vi "ConduccionTermica.vi"() -> ()   [LabVIEW 2024]
uses:
  <vilib>/express/express shared/transition.llb/Dynamic To Waveform Array.vi
  <vilib>/express/express signal manip/GetorSetDDTAttributes/Set DDT Attributes/SetT0.vi
  <vilib>/express/express shared/transition.llb/Waveform Array To Dynamic.vi
  <vilib>/express/express signal manip/GetorSetDDTAttributes/Set DDT Attributes/Set DDT Properties.xnode
  <instrlib>/Arduino UNO/Arduino UNO.lvlib
panel:
  out "Sensor V 2":dbl
  out "Sensor 2":string
  out "Temperatura V 5":dbl
  out "Temperatura 5":string
  out "Temperatura V 4":dbl
  out "Temperatura 4":string
  out "Sensor V 1":dbl
  out "Sensor 1":string
  in  "COM 2":refnum<visa-resource-name>
  out "Temperatura V 3":dbl
  out "Temperatura V 2":dbl
  out "Temperatura V 1":dbl
  in  "stop":bool
  in  "COM 1":refnum<visa-resource-name>
  out "Temperatura 3":string
  out "Temperatura 2":string
  out "Temperatura 1":string
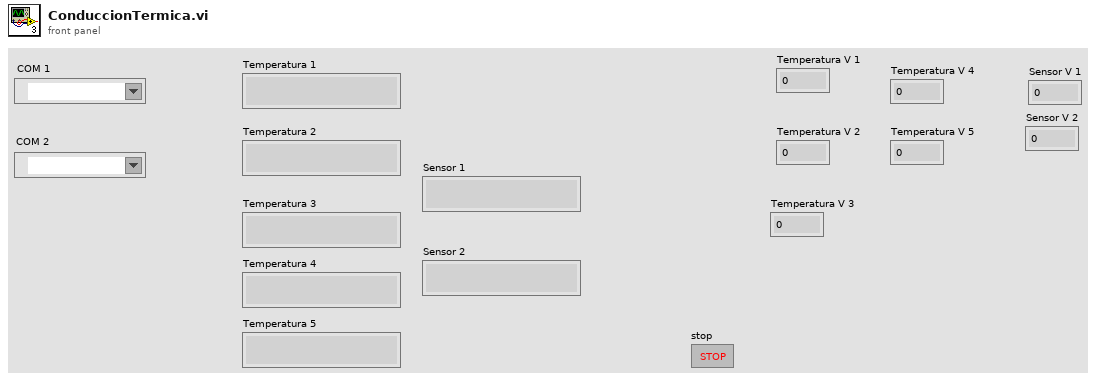
[diagram p1: front panel]
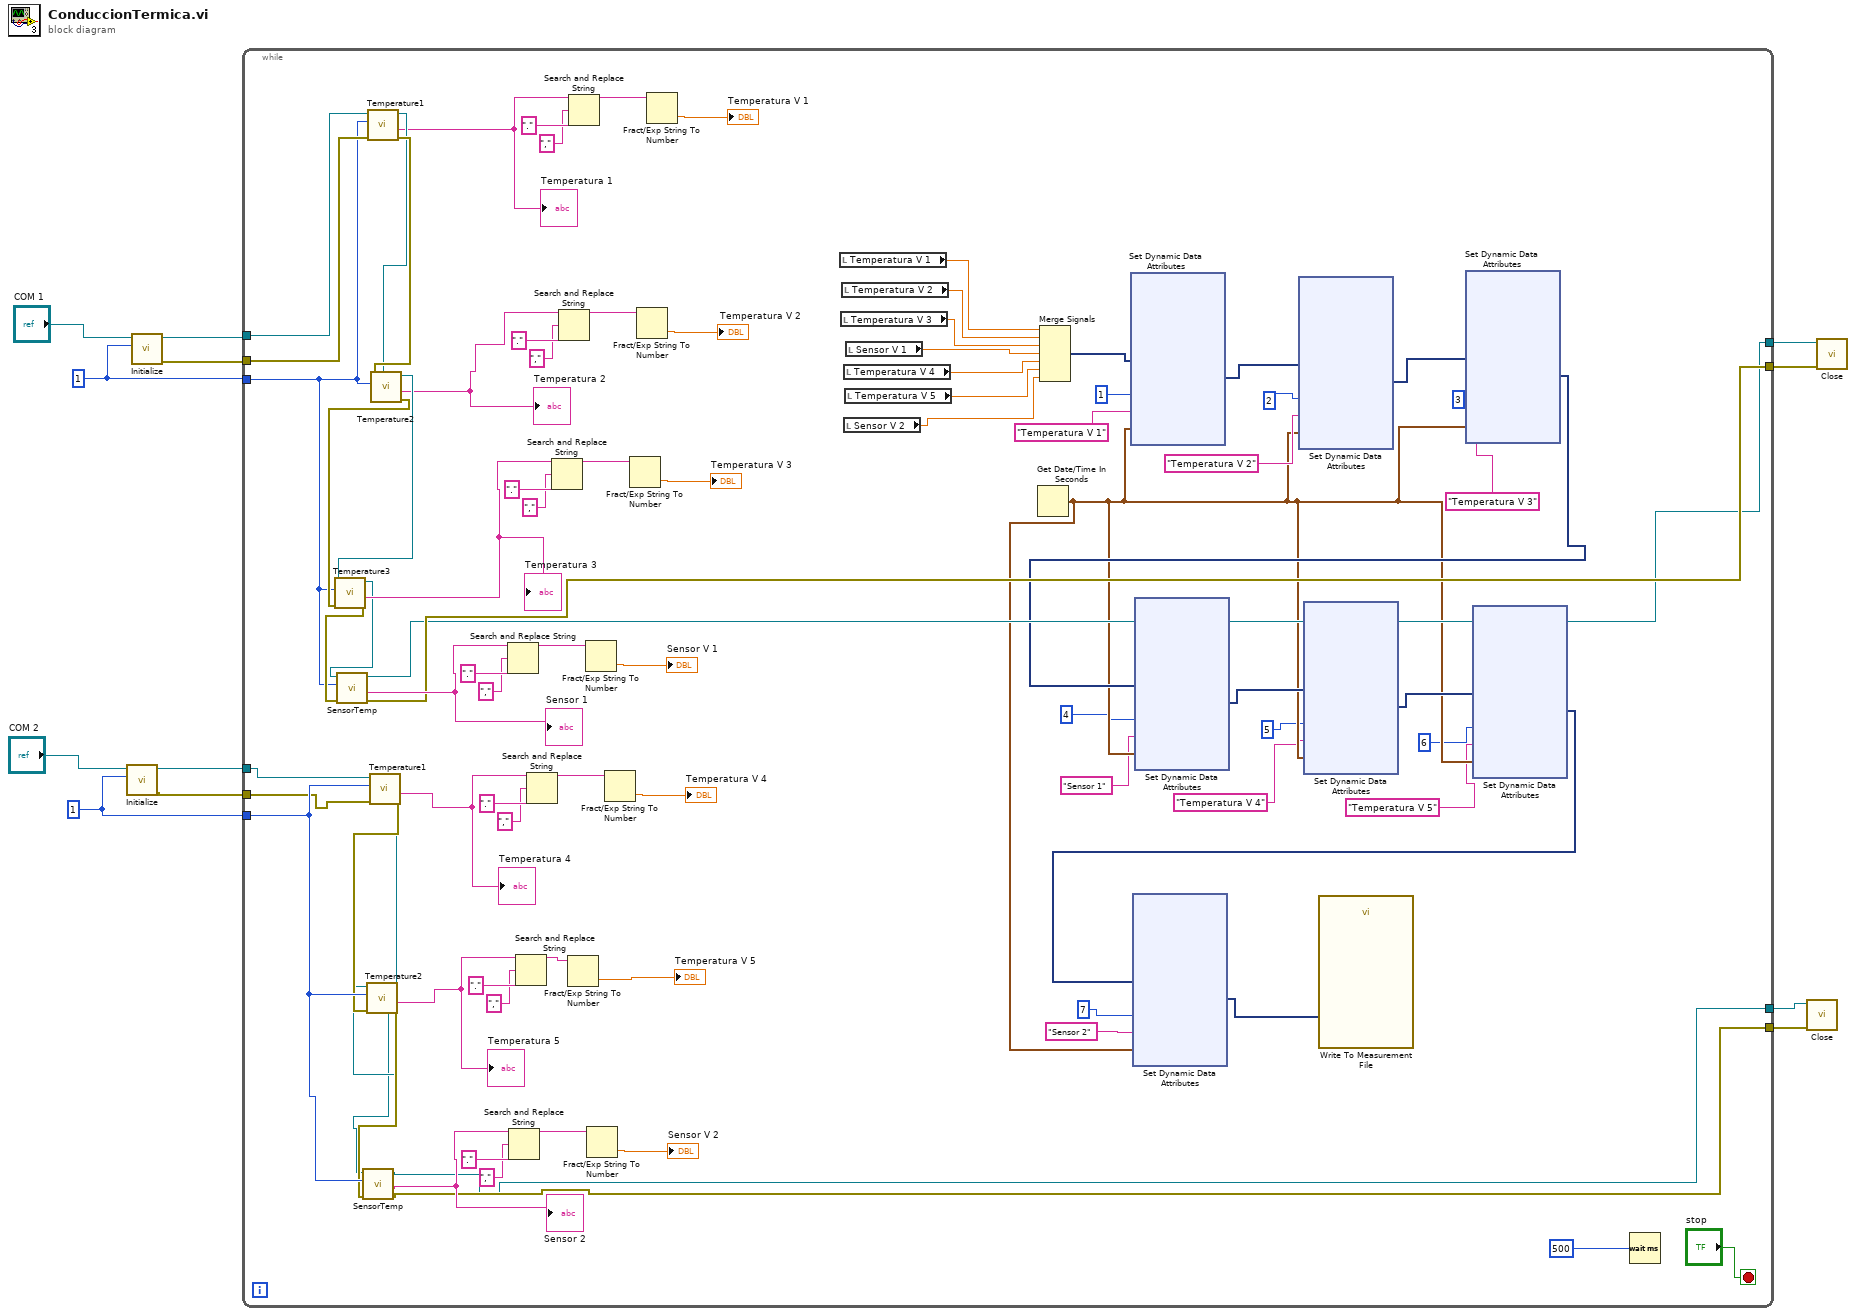
[diagram p0: block diagram]
diagram:
  w5 = 1
  w9 = 1
  n1 = call <instrlib>:"Initialize.vi"("Address"=w5, "VISA resource name"="COM 2") -> ("error IO"=w4:errorcluster, "VISA resource name out"=w3:refnum<visa-resource-name>)  [unwired: 7 in, 1 out]
  n2 = call <instrlib>:"Initialize.vi"("Address"=w9, "VISA resource name"="COM 1") -> ("error IO"=w10:errorcluster, "VISA resource name out"=w11:refnum<visa-resource-name>)  [unwired: 7 in, 1 out]
  n3 = while {
    tunnel: w11 -> [w69]
    tunnel: w10 -> [w68]
    tunnel: w9 -> [w62]
    tunnel: [w55] -> w8
    tunnel: [w56] -> w7
    tunnel: w5 -> [w52]
    tunnel: w4 -> [w51]
    tunnel: w3 -> [w53]
    tunnel: [w31] -> w1
    tunnel: [w30] -> w2
    stop <- "stop" stop-if-true
    n4 = call <instrlib>:"Temperature1.vi"("error in (no error)"=w68, "Address"=w62, "VISA resource name"=w69) -> ("error IO"=w67:errorcluster, "Pressure"=w65:string, "VISA resource name out"=w66:refnum<visa-resource-name>)  [unwired: 6 in]
    "Temperatura 1" <- w65
    n5 = call <instrlib>:"Temperature1.vi"("error in (no error)"=w51, "Address"=w52, "VISA resource name"=w53) -> ("error IO"=w50:errorcluster, "Pressure"=w42:string, "VISA resource name out"=w48:refnum<visa-resource-name>)  [unwired: 6 in]
    "Temperatura 4" <- w42
    n6 = call <instrlib>:"Temperature2.vi"("error in (no error)"=w50, "Address"=w52, "VISA resource name"=w48) -> ("error IO"=w49:errorcluster, "Pressure"=w37:string, "VISA resource name out"=w47:refnum<visa-resource-name>)  [unwired: 6 in]
    "Temperatura 5" <- w37
    n7 = call <instrlib>:"SensorTemp.vi"("error in (no error)"=w49, "Address"=w52, "VISA resource name"=w47) -> ("error IO"=w31:errorcluster, "Pressure"=w32:string, "VISA resource name out"=w30:refnum<visa-resource-name>)  [unwired: 6 in]
    "Sensor 2" <- w32
    n8 = call <instrlib>:"Temperature2.vi"("error in (no error)"=w67, "Address"=w62, "VISA resource name"=w66) -> ("error IO"=w70:errorcluster, "Pressure"=w89:string, "VISA resource name out"=w98:refnum<visa-resource-name>)  [unwired: 6 in]
    "Temperatura 2" <- w89
    n9 = call <instrlib>:"Temperature3.vi"("error in (no error)"=w70, "Address"=w62, "VISA resource name"=w98) -> ("error IO"=w63:errorcluster, "Pressure"=w84:string, "VISA resource name out"=w64:refnum<visa-resource-name>)  [unwired: 6 in]
    "Temperatura 3" <- w84
    n10 = call <instrlib>:"SensorTemp.vi"("error in (no error)"=w63, "Address"=w62, "VISA resource name"=w64) -> ("error IO"=w56:errorcluster, "Pressure"=w57:string, "VISA resource name out"=w55:refnum<visa-resource-name>)  [unwired: 6 in]
    "Sensor 1" <- w57
    n11 = Search and Replace String(input string=w57, search string=".", replace string=",") -> (result string=w59:string)  [unwired: 5 in, 3 out]
    n12 = Search and Replace String(input string=w32, search string=".", replace string=",") -> (result string=w34:string)  [unwired: 5 in, 3 out]
    n13 = Search and Replace String(input string=w37, search string=".", replace string=",") -> (result string=w39:string)  [unwired: 5 in, 3 out]
    n14 = Search and Replace String(input string=w42, search string=".", replace string=",") -> (result string=w44:string)  [unwired: 5 in, 3 out]
    n15 = Search and Replace String(input string=w84, search string=".", replace string=",") -> (result string=w86:string)  [unwired: 5 in, 3 out]
    n16 = Search and Replace String(input string=w89, search string=".", replace string=",") -> (result string=w91:string)  [unwired: 5 in, 3 out]
    n17 = Fract/Exp String To Number(string=w39) -> (number=→"Temperatura V 5":dbl)  [unwired: 3 in, 1 out]
    n18 = Search and Replace String(input string=w65, search string=".", replace string=",") -> (result string=w95:string)  [unwired: 5 in, 3 out]
    n19 = Fract/Exp String To Number(string=w59) -> (number=→"Sensor V 1":dbl)  [unwired: 3 in, 1 out]
    n20 = Fract/Exp String To Number(string=w34) -> (number=→"Sensor V 2":dbl)  [unwired: 3 in, 1 out]
    n21 = Fract/Exp String To Number(string=w44) -> (number=→"Temperatura V 4":dbl)  [unwired: 3 in, 1 out]
    n22 = Fract/Exp String To Number(string=w86) -> (number=→"Temperatura V 3":dbl)  [unwired: 3 in, 1 out]
    n23 = Fract/Exp String To Number(string=w91) -> (number=→"Temperatura V 2":dbl)  [unwired: 3 in, 1 out]
    n24 = Fract/Exp String To Number(string=w95) -> (number=→"Temperatura V 1":dbl)  [unwired: 3 in, 1 out]
    n25 = local read "Temperatura V 1"() -> (w82:dbl)
    n26 = local read "Temperatura V 3"() -> (w80:dbl)
    n27 = local read "Temperatura V 2"() -> (w81:dbl)
    n28 = local read "Temperatura V 4"() -> (w29:dbl)
    n29 = local read "Sensor V 2"() -> (w27:dbl)
    n30 = local read "Temperatura V 5"() -> (w28:dbl)
    n31 = local read "Sensor V 1"() -> (w54:dbl)
    n32 = Get Date/Time In Seconds() -> (seconds since 1Jan1904=w21:timestamp)
    n33 = Merge Signals(w82, w81, w80, w54, w29, w28, w27) -> (w79:dynamicdata)
    n34 = xnode "Set Dynamic Data Attributes"("Signals In"=w79, "Signal Index"=1, "Signal Name"="Temperatura V 1", "Timestamp"=w21) -> ("Signals Out"=w78:dynamicdata)  [unwired: 1 in, 1 out]
    n35 = xnode "Set Dynamic Data Attributes"("Signals In"=w78, "Signal Index"=2, "Signal Name"="Temperatura V 2", "Timestamp"=w21) -> ("Signals Out"=w77:dynamicdata)  [unwired: 1 in, 1 out]
    n36 = xnode "Set Dynamic Data Attributes"("Signals In"=w77, "Signal Index"=3, "Signal Name"="Temperatura V 3", "Timestamp"=w21) -> ("Signals Out"=w26:dynamicdata)  [unwired: 1 in, 1 out]
    n37 = xnode "Set Dynamic Data Attributes"("Signals In"=w26, "Signal Index"=4, "Signal Name"="Sensor 1", "Timestamp"=w21) -> ("Signals Out"=w25:dynamicdata)  [unwired: 1 in, 1 out]
    n38 = xnode "Set Dynamic Data Attributes"("Signals In"=w25, "Signal Index"=5, "Signal Name"="Temperatura V 4", "Timestamp"=w21) -> ("Signals Out"=w24:dynamicdata)  [unwired: 1 in, 1 out]
    n39 = xnode "Set Dynamic Data Attributes"("Signals In"=w24, "Signal Index"=6, "Signal Name"="Temperatura V 5", "Timestamp"=w21) -> ("Signals Out"=w23:dynamicdata)  [unwired: 1 in, 1 out]
    n40 = xnode "Set Dynamic Data Attributes"("Signals In"=w23, "Signal Index"=7, "Signal Name"="Sensor 2", "Timestamp"=w21) -> ("Signals Out"=w22:dynamicdata)  [unwired: 1 in, 1 out]
    n41 = call "Write To Measurement File"("Signals"=w22) -> ()  [unwired: 16 in, 3 out]
    n42 = Wait (ms)(milliseconds to wait=u32 500) -> ()  [unwired: 1 out]
  }
  n43 = call <instrlib>:"Close.vi"("error in (no error)"=w1, "VISA resource name"=w2) -> ()  [unwired: 9 in, 1 out]
  n44 = call <instrlib>:"Close.vi"("error in (no error)"=w7, "VISA resource name"=w8) -> ()  [unwired: 9 in, 1 out]
